vi "MPC-200 trajectory-multi.vi"() -> ()   [LabVIEW 2013]
panel:
  in  "Trace Ok?":bool
  in  "Number of passes":i32=4
  out "DATA DISPLAY 4":cluster{dbl[], dbl[]}(graph)
  out "DATA DISPLAY 3":cluster{dbl[], dbl[]}(graph)
  out "Time per line (ms) 2":i32
  out "DATA DISPLAY 2":cluster{dbl[], dbl[]}(graph)
  out "start position (um)":dbl[](array[numeric])
  out "end position (um)":dbl[](array[numeric])
  in  "Input Start Position":bool
  in  "Input End Position":bool
  out "DATA DISPLAY":cluster{dbl[], dbl[]}(graph)
  out "Time per line (ms)":i32
  in  "Step  size (um)":dbl=150.0
  in  "Start?":bool
  in  "Stop?":bool
  in  "error in (no error)":errorcluster
  out "sutter connection checked":bool
  out "Initial position":dbl[](array[numeric])
  out "error out":errorcluster
  in  "sutter serial port connetion":string(combo)="COM5"
  # "x in um"
  # "y in  um"
  # "z in  um"
  # "x in um"
  # "x in um"
  # "y in  um"
  # "y in  um"
  # "z in  um"
  # "z in  um"
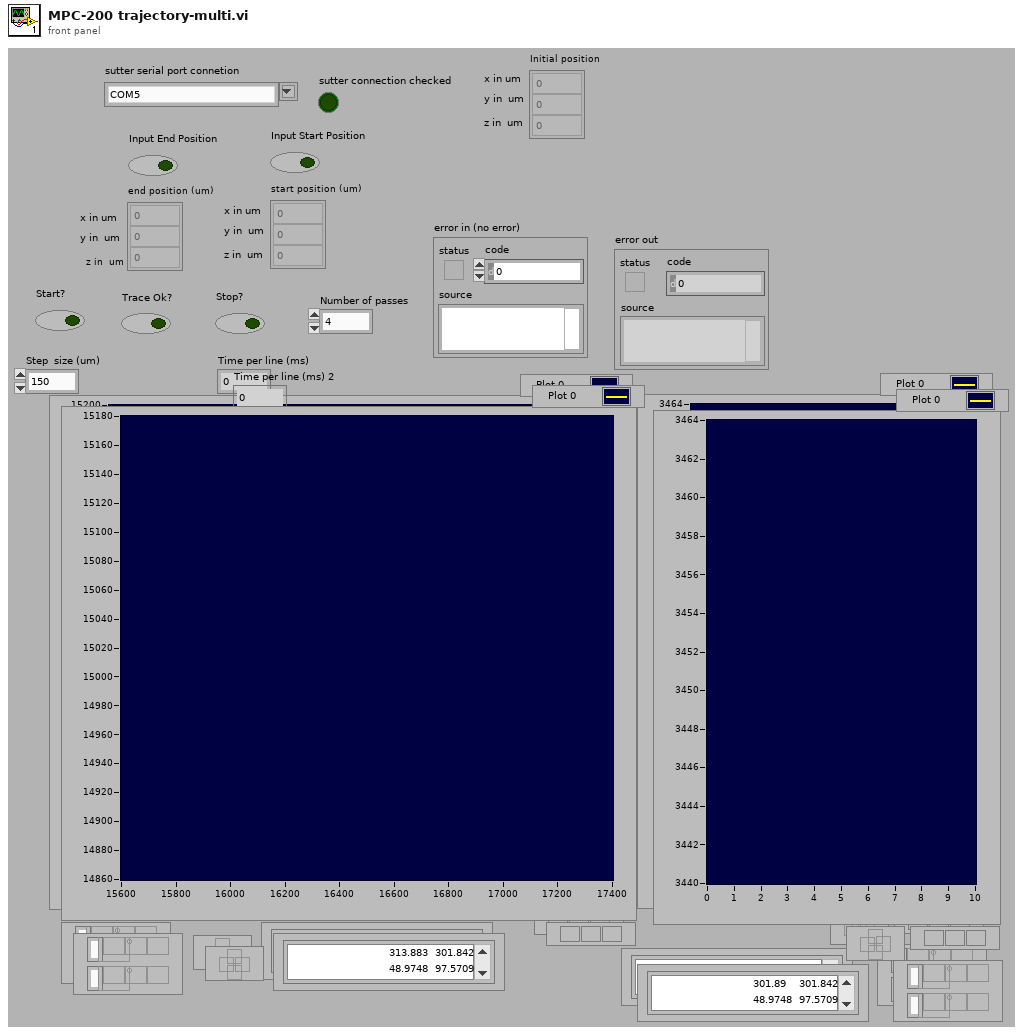
[diagram p1: front panel]
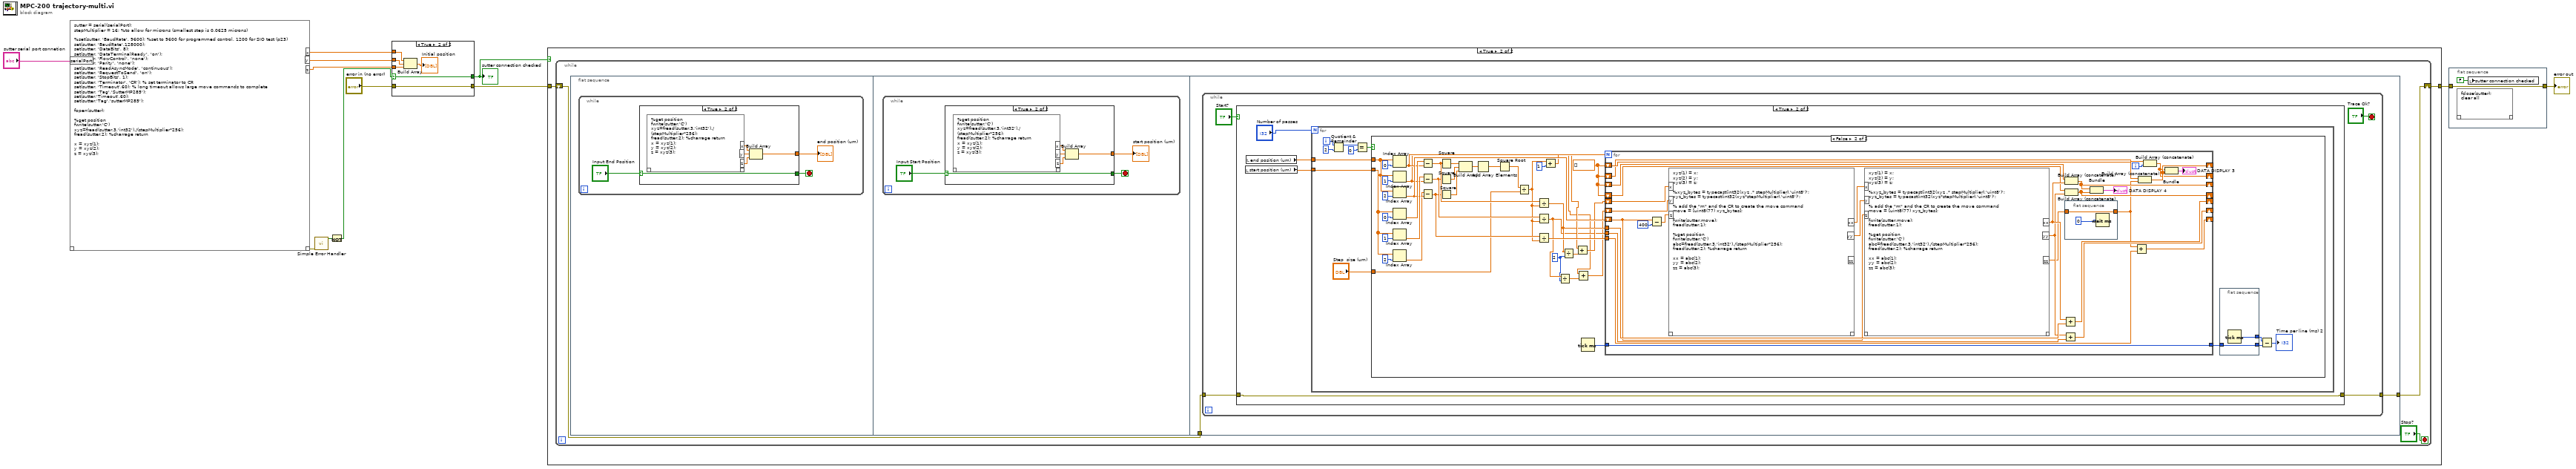
[diagram p0: block diagram]
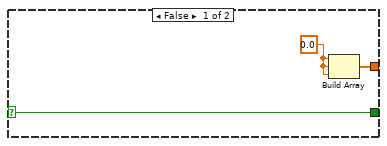
[diagram p3: hidden frame]
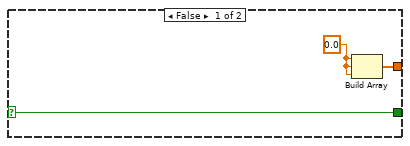
[diagram p4: hidden frame]
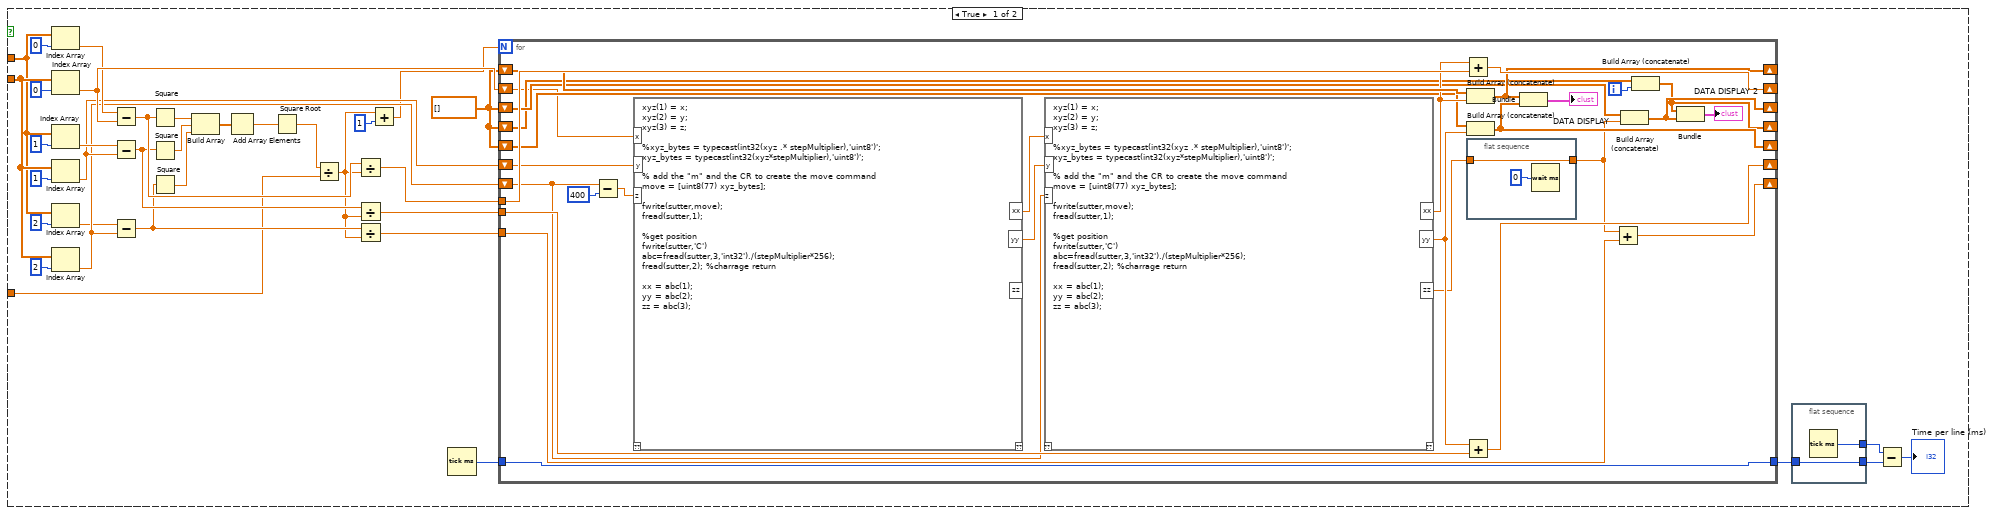
[diagram p6: hidden frame]
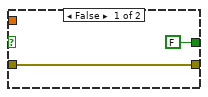
[diagram p7: hidden frame]
diagram:
  n1 = script code="sutter = serial(serialPort);\nstepMultiplier = 16; %to allow for microns (smallest step is 0.0625 microns)\n\n%set(sutter, 'BaudRate', 9600); %set to 9600 for programmed control, 1200 for SIO test (p23)\nset(sutter, 'BaudRate',128000);\nset(sutter, 'DataBits', 8);\nset(sutter, 'DataTerminalReady', 'on');\nset(sutter, 'FlowControl', 'none');\nset(sutter, 'Parity', 'none');\nset(sutter, 'ReadAsyncMode', 'continuous');\nset(sutter, 'RequestToSend', 'on');\nset(sutter, 'StopBits', 1);\nset(sutter, 'Terminator', 'CR'); % set terminator to CR\nset(sutter, 'Timeout',60); % long timeout allows large move commands to complete\nset(sutter, 'Tag','SutterMP285');\nset(sutter,'Timeout',60);\nset(sutter,'Tag','sutterMP285');\n\nfopen(sutter);\n\n%get position\nfwrite(sutter,'C')\nxyz=fread(sutter,3,'int32')./(stepMultiplier*256);\nfread(sutter,2); %charrage return\n\nx = xyz(1);\ny = xyz(2);\nz = xyz(3);"("serialPort"="sutter serial port connetion") -> ("??"=w9:errorcluster, "x"=w12:dbl, "y"=w11:dbl, "z"=w10:dbl)  [unwired: 1 in]
  n2 = call <vilib>:"Simple Error Handler.vi"("error in (no error)"=w9) -> ("error?"=w7:bool)  [unwired: 4 in, 4 out]
  n3 = Not(x=w7) -> (.not. x?=w8:bool)
  n4 = case shown="True" w8 {
    selector: w8 -> [_ w17]
    tunnel: w12 -> [_ w20]
    tunnel: w11 -> [_ w19]
    tunnel: w10 -> [_ w18]
    tunnel: [FALSE w17] -> w3
    tunnel: "error in (no error)" -> [w13 w15]
    tunnel: [w13 w15] -> w4
    frame False {
    }
    frame True {
      n5 = Build Array(w20, w19, w18) -> (→"Initial position":dbl[])
    }
  }
  "sutter connection checked" <- w3
  n6 = case shown="True" w3 {
    tunnel: w4 -> [w21 w23]
    tunnel: [w21 w22] -> w2
    frame False {
    }
    frame True {
      n7 = while {
        shift-right: [w25] -> w22
        shift-left: w23 -> [w26]
        stop <- "Stop?" stop-if-true
        n8 = flat-sequence {
          tunnel: w26 -> [w50]
          tunnel: [w49] -> w25
          frame #0 {
            n9 = while {
              stop <- w28 stop-if-true
              n10 = case shown="True" "Input End Position" {
                selector: "Input End Position" -> [w32 w37]
                tunnel: [w32 w37] -> w28
                tunnel: [w31 w33] -> w27
                frame False {
                  w30 = 0.0
                  n11 = Build Array(w30, w30, w30) -> (w31:dbl[])
                }
                frame True {
                  n12 = script code="%get position\nfwrite(sutter,'C')\nxyz=fread(sutter,3,'int32')./(stepMultiplier*256);\nfread(sutter,2); %charrage return\nx = xyz(1);\ny = xyz(2);\nz = xyz(3);"() -> ("x"=w36:dbl, "y"=w35:dbl, "z"=w34:dbl)  [unwired: 1 in, 1 out]
                  n13 = Build Array(w36, w35, w34) -> (w33:dbl[])
                }
              }
              "end position (um)" <- w27
            }
          }
          frame #1 {
            n14 = while {
              stop <- w39 stop-if-true
              n15 = case shown="True" "Input Start Position" {
                selector: "Input Start Position" -> [w43 w48]
                tunnel: [w43 w48] -> w39
                tunnel: [w41 w44] -> w38
                frame False {
                  w42 = 0.0
                  n16 = Build Array(w42, w42, w42) -> (w41:dbl[])
                }
                frame True {
                  n17 = script code="%get position\nfwrite(sutter,'C')\nxyz=fread(sutter,3,'int32')./(stepMultiplier*256);\nfread(sutter,2); %charrage return\nx = xyz(1);\ny = xyz(2);\nz = xyz(3);"() -> ("x"=w47:dbl, "y"=w46:dbl, "z"=w45:dbl)  [unwired: 1 in, 1 out]
                  n18 = Build Array(w47, w46, w45) -> (w44:dbl[])
                }
              }
              "start position (um)" <- w38
            }
          }
          frame #2 {
            n19 = while {
              tunnel: w50 -> [w54]
              tunnel: [w53] -> w49
              stop <- "Trace Ok?" stop-if-true
              n20 = case shown="True" "Start?" {
                tunnel: [w55 w59] -> w53
                tunnel: w54 -> [w55 w59]
                frame False {
                }
                frame True {
                  n21 = local read "start position (um)"() -> (w58:dbl[])
                  n22 = local read "end position (um)"() -> (w57:dbl[])
                  n23 = for {
                    N: "Number of passes" -> [_]
                    tunnel: w57 -> [w66]
                    tunnel: w58 -> [w67]
                    i -> [w61]
                    n24 = Quotient & Remainder(x=w61, y=2) -> (x-y*floor(x/y)=w64:i32)  [unwired: 1 out]
                    n25 = Equal?(x=w64, y=0) -> (x = y?=w62:bool)
                    n26 = case shown="False" w62 {
                      tunnel: w67 -> [w71 w147]
                      tunnel: w66 -> [w70 w148]
                      tunnel: "Step  size (um)" -> [w68 w146]
                      frame True {
                        w69 = dbl[] []
                        n27 = Index Array(array=w70, index=0) -> (element=w79:dbl)
                        n28 = Index Array(array=w71, index=0) -> (element=w80:dbl)
                        n29 = Index Array(array=w70, index=1) -> (element=w78:dbl)
                        n30 = Index Array(array=w71, index=1) -> (element=w77:dbl)
                        n31 = Index Array(array=w70, index=2) -> (element=w75:dbl)
                        n32 = Index Array(array=w71, index=2) -> (element=w76:dbl)
                        n33 = Subtract(x=w79, y=w80) -> (x-y=w90:dbl)
                        n34 = Subtract(x=w78, y=w77) -> (x-y=w89:dbl)
                        n35 = Subtract(x=w75, y=w76) -> (x-y=w88:dbl)
                        n36 = Square(x=w90) -> (x^2=w96:dbl)
                        n37 = Square(x=w89) -> (x^2=w95:dbl)
                        n38 = Square(x=w88) -> (x^2=w94:dbl)
                        n39 = Build Array(w96, w95, w94) -> (w93:dbl[])
                        n40 = Add Array Elements(numeric array=w93) -> (sum=w92:dbl)
                        n41 = Square Root(x=w92) -> (sqrt(x)=w91:dbl)
                        n42 = Divide(x=w91, y=w68) -> (x/y=w72:dbl)
                        n43 = Divide(x=w90, y=w72) -> (x/y=w87:dbl)
                        n44 = Divide(x=w89, y=w72) -> (x/y=w86:dbl)
                        n45 = Divide(x=w88, y=w72) -> (x/y=w85:dbl)
                        n46 = Add(x=w72, y=1) -> (x+y=w73:dbl)
                        n47 = Tick Count (ms)() -> (millisecond timer value=w103:u32)
                        n48 = for {
                          N: w73 -> [_]
                          tunnel: w103 -> [w130]
                          shift-right: [w133] -> _
                          shift-left: w80 -> [w114]
                          shift-right: [w123] -> _
                          shift-left: w76 -> [w108]
                          shift-right: [w122] -> _
                          shift-left: w77 -> [w112]
                          tunnel: w87 -> [w134]
                          tunnel: w86 -> [w132]
                          tunnel: w85 -> [w131]
                          tunnel: [w130] -> w84
                          shift-right: [w121] -> _
                          shift-left: w69 -> [w129]
                          shift-right: [w124] -> _
                          shift-left: w69 -> [w127]
                          shift-right: [w118] -> _
                          shift-left: w69 -> [w120]
                          shift-right: [w115] -> _
                          shift-left: w69 -> [w117]
                          i -> [w116]
                          n49 = Subtract(x=w108, y=400) -> (x-y=w109:dbl)
                          n50 = script code="xyz(1) = x;\nxyz(2) = y;\nxyz(3) = z;\n\n%xyz_bytes = typecast(int32(xyz .* stepMultiplier),'uint8')';\nxyz_bytes = typecast(int32(xyz*stepMultiplier),'uint8')';\n\n% add the \"m\" and the CR to create the move command\nmove = [uint8(77) xyz_bytes];\n\nfwrite(sutter,move);\nfread(sutter,1);\n\n%get position\nfwrite(sutter,'C')\nabc=fread(sutter,3,'int32')./(stepMultiplier*256);\nfread(sutter,2); %charrage return\n\nxx = abc(1);\nyy = abc(2);\nzz = abc(3);"("x"=w114, "y"=w112, "z"=w109) -> ("xx"=w113:dbl, "yy"=w111:dbl)  [unwired: 1 in, 2 out]
                          n51 = script code="xyz(1) = x;\nxyz(2) = y;\nxyz(3) = z;\n\n%xyz_bytes = typecast(int32(xyz .* stepMultiplier),'uint8')';\nxyz_bytes = typecast(int32(xyz*stepMultiplier),'uint8')';\n\n% add the \"m\" and the CR to create the move command\nmove = [uint8(77) xyz_bytes];\n\nfwrite(sutter,move);\nfread(sutter,1);\n\n%get position\nfwrite(sutter,'C')\nabc=fread(sutter,3,'int32')./(stepMultiplier*256);\nfread(sutter,2); %charrage return\n\nxx = abc(1);\nyy = abc(2);\nzz = abc(3);"("x"=w113, "y"=w111, "z"=w108) -> ("zz"=w107:dbl, "xx"=w128:dbl, "yy"=w126:dbl)  [unwired: 1 in, 1 out]
                          n52 = Add(x=w128, y=w134) -> (x+y=w133:dbl)
                          n53 = Add(x=w126, y=w132) -> (x+y=w122:dbl)
                          n54 = Build Array (concatenate)(w129, w128) -> (w121:dbl[])
                          n55 = Build Array (concatenate)(w127, w126) -> (w124:dbl[])
                          n56 = flat-sequence {
                            tunnel: w107 -> [w135]
                            tunnel: [w135] -> w106
                            frame #0 {
                              n57 = Wait (ms)(milliseconds to wait=0) -> ()  [unwired: 1 out]
                            }
                          }
                          n58 = Bundle(w121, w124) -> (→"DATA DISPLAY":cluster{dbl[], dbl[]})  [unwired: 1 in]
                          n59 = Add(x=w106, y=w131) -> (x+y=w123:dbl)
                          n60 = Build Array (concatenate)(w120, w106) -> (w118:dbl[])
                          n61 = Build Array (concatenate)(w117, w116) -> (w115:dbl[])
                          n62 = Bundle(w115, w118) -> (→"DATA DISPLAY 2":cluster{dbl[], dbl[]})  [unwired: 1 in]
                        }
                        n63 = flat-sequence {
                          tunnel: [w105] -> w83
                          tunnel: w84 -> [w105]
                          tunnel: [w104] -> w82
                          frame #0 {
                            n64 = Tick Count (ms)() -> (millisecond timer value=w104:u32)
                          }
                        }
                        n65 = Subtract(x=w82, y=w83) -> (x-y=→"Time per line (ms)":u32)
                      }
                      frame False {
                        w140 = 2
                        w149 = dbl[] []
                        n66 = Index Array(array=w148, index=0) -> (element=w145:dbl)
                        n67 = Index Array(array=w148, index=1) -> (element=w138:dbl)
                        n68 = Index Array(array=w148, index=2) -> (element=w154:dbl)
                        n69 = Index Array(array=w147, index=0) -> (element=w156:dbl)
                        n70 = Index Array(array=w147, index=1) -> (element=w155:dbl)
                        n71 = Index Array(array=w147, index=2) -> (element=w153:dbl)
                        n72 = Subtract(x=w156, y=w145) -> (x-y=w164:dbl)
                        n73 = Subtract(x=w155, y=w138) -> (x-y=w163:dbl)
                        n74 = Subtract(x=w153, y=w154) -> (x-y=w162:dbl)
                        n75 = Square(x=w164) -> (x^2=w170:dbl)
                        n76 = Square(x=w163) -> (x^2=w169:dbl)
                        n77 = Square(x=w162) -> (x^2=w168:dbl)
                        n78 = Build Array(w170, w169, w168) -> (w167:dbl[])
                        n79 = Add Array Elements(numeric array=w167) -> (sum=w166:dbl)
                        n80 = Square Root(x=w166) -> (sqrt(x)=w165:dbl)
                        n81 = Divide(x=w165, y=w146) -> (x/y=w150:dbl)
                        n82 = Divide(x=w164, y=w150) -> (x/y=w144:dbl)
                        n83 = Divide(x=w163, y=w150) -> (x/y=w141:dbl)
                        n84 = Divide(x=w162, y=w150) -> (x/y=w161:dbl)
                        n85 = Add(x=w150, y=1) -> (x+y=w151:dbl)
                        n86 = Divide(x=w141, y=w140) -> (x/y=w139:dbl)
                        n87 = Divide(x=w144, y=w140) -> (x/y=w143:dbl)
                        n88 = Add(x=w145, y=w143) -> (x+y=w142:dbl)
                        n89 = Add(x=w138, y=w139) -> (x+y=w137:dbl)
                        n90 = Tick Count (ms)() -> (millisecond timer value=w177:u32)
                        n91 = for {
                          N: w151 -> [_]
                          tunnel: w177 -> [w204]
                          shift-right: [w207] -> _
                          shift-left: w142 -> [w188]
                          shift-right: [w197] -> _
                          shift-left: w154 -> [w182]
                          shift-right: [w196] -> _
                          shift-left: w137 -> [w186]
                          tunnel: w144 -> [w208]
                          tunnel: w141 -> [w206]
                          tunnel: w161 -> [w205]
                          tunnel: [w204] -> w160
                          shift-right: [w195] -> _
                          shift-left: w149 -> [w203]
                          shift-right: [w198] -> _
                          shift-left: w149 -> [w201]
                          shift-right: [w192] -> _
                          shift-left: w149 -> [w194]
                          shift-right: [w189] -> _
                          shift-left: w149 -> [w191]
                          i -> [w190]
                          n92 = Subtract(x=w182, y=400) -> (x-y=w183:dbl)
                          n93 = script code="xyz(1) = x;\nxyz(2) = y;\nxyz(3) = z;\n\n%xyz_bytes = typecast(int32(xyz .* stepMultiplier),'uint8')';\nxyz_bytes = typecast(int32(xyz*stepMultiplier),'uint8')';\n\n% add the \"m\" and the CR to create the move command\nmove = [uint8(77) xyz_bytes];\n\nfwrite(sutter,move);\nfread(sutter,1);\n\n%get position\nfwrite(sutter,'C')\nabc=fread(sutter,3,'int32')./(stepMultiplier*256);\nfread(sutter,2); %charrage return\n\nxx = abc(1);\nyy = abc(2);\nzz = abc(3);"("x"=w188, "y"=w186, "z"=w183) -> ("xx"=w187:dbl, "yy"=w185:dbl)  [unwired: 1 in, 2 out]
                          n94 = script code="xyz(1) = x;\nxyz(2) = y;\nxyz(3) = z;\n\n%xyz_bytes = typecast(int32(xyz .* stepMultiplier),'uint8')';\nxyz_bytes = typecast(int32(xyz*stepMultiplier),'uint8')';\n\n% add the \"m\" and the CR to create the move command\nmove = [uint8(77) xyz_bytes];\n\nfwrite(sutter,move);\nfread(sutter,1);\n\n%get position\nfwrite(sutter,'C')\nabc=fread(sutter,3,'int32')./(stepMultiplier*256);\nfread(sutter,2); %charrage return\n\nxx = abc(1);\nyy = abc(2);\nzz = abc(3);"("x"=w187, "y"=w185, "z"=w182) -> ("zz"=w181:dbl, "xx"=w202:dbl, "yy"=w200:dbl)  [unwired: 1 in, 1 out]
                          n95 = Add(x=w202, y=w208) -> (x+y=w207:dbl)
                          n96 = Add(x=w200, y=w206) -> (x+y=w196:dbl)
                          n97 = Build Array (concatenate)(w203, w202) -> (w195:dbl[])
                          n98 = Build Array (concatenate)(w201, w200) -> (w198:dbl[])
                          n99 = flat-sequence {
                            tunnel: w181 -> [w209]
                            tunnel: [w209] -> w180
                            frame #0 {
                              n100 = Wait (ms)(milliseconds to wait=0) -> ()  [unwired: 1 out]
                            }
                          }
                          n101 = Bundle(w195, w198) -> (→"DATA DISPLAY 4":cluster{dbl[], dbl[]})  [unwired: 1 in]
                          n102 = Add(x=w180, y=w205) -> (x+y=w197:dbl)
                          n103 = Build Array (concatenate)(w194, w180) -> (w192:dbl[])
                          n104 = Build Array (concatenate)(w191, w190) -> (w189:dbl[])
                          n105 = Bundle(w189, w192) -> (→"DATA DISPLAY 3":cluster{dbl[], dbl[]})  [unwired: 1 in]
                        }
                        n106 = flat-sequence {
                          tunnel: [w179] -> w159
                          tunnel: w160 -> [w179]
                          tunnel: [w178] -> w158
                          frame #0 {
                            n107 = Tick Count (ms)() -> (millisecond timer value=w178:u32)
                          }
                        }
                        n108 = Subtract(x=w158, y=w159) -> (x-y=→"Time per line (ms) 2":u32)
                      }
                    }
                  }
                }
              }
            }
          }
        }
      }
    }
  }
  n109 = flat-sequence {
    tunnel: w2 -> [w212]
    tunnel: [w212] -> w1
    frame #0 {
      n110 = script code="fclose(sutter);\nclear all"() -> ()  [unwired: 1 in, 1 out]
      n111 = local write "sutter connection checked"(FALSE) -> ()
    }
  }
  "error out" <- w1
